vi "Read Process State Data.vi"(8 "error in (no error)":errorcluster, 11 "Laser Controller in":refnum<class "Laser Controller.lvclass">) -> (0 "error out":errorcluster, 2 "Process State Data":refnum<data-value>, 3 "Laser Controller out":refnum<class "Laser Controller.lvclass">)   [LabVIEW 2022 SP3, in "Laser Controller.lvclass"]
uses:
  Laser Controller.lvclass
  XY Stage/Process Actor/Process Framework/Process State Data/Process State Data.lvclass
  Laser Controller.lvclass/Laser Controller.ctl
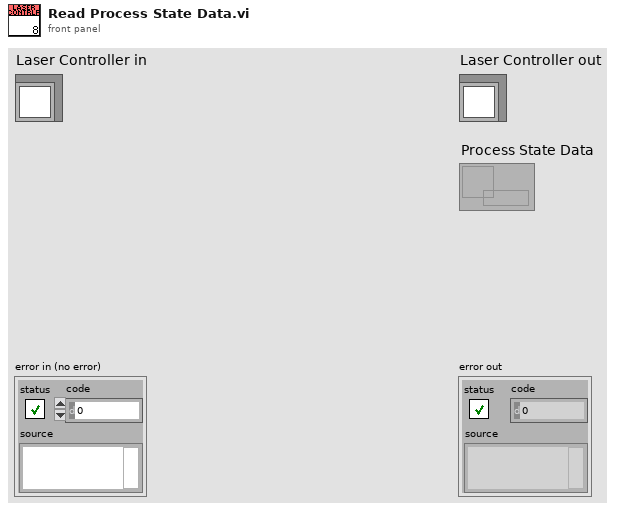
[diagram p1: front panel]
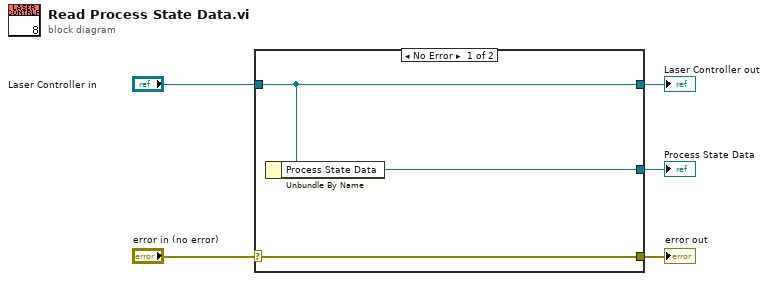
[diagram p0: block diagram]
diagram:
  n1 = case shown="No Error" "error in (no error)" {
    selector: "error in (no error)" -> [w8 w9]
    tunnel: [w8 w9] -> w4
    tunnel: [w7 w10] -> w2
    tunnel: "Laser Controller in" -> [w7 w10]
    tunnel: [w6 _] -> w1
    frame No Error {
      n2 = Unbundle By Name(w7) -> ("Process State Data"=w6:refnum<data-value>)
    }
    frame Error {
    }
  }
  "error out" <- w4
  "Laser Controller out" <- w2
  "Process State Data" <- w1
